vi "Main.vi"   [LabVIEW 2021]
uses:
  Dev Actor/Dev Actor/Dev Actor.lvclass
  C:/git/jettl/src/LVCAM/LVCAM/Actor/Actor.lvclass
  src/LVCAM/LVCAM/Self Actor/Self Actor.lvclass
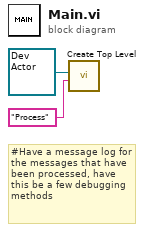
[diagram p0: block diagram]
diagram:
  # "#Have a message log for the messages that have been processed, have this be a few debugging methods"
  n1 = call "Create Top Level.vi"("Alias"="Process", "Actor"=refnum<class "Dev Actor.lvclass"> refnum ("Process.lvlib:Process.lvclass")) -> ()  [unwired: 10 in]
